vi "Get_user_id.vi"(8 "error in":errorcluster, 11 "Device In":T1) -> (0 "error out":errorcluster, 1 "id":string, 2 "Comm":T2, 3 "Device Out":T1)   [LabVIEW 2019]
uses:
  <userlib>/IoT Devices/_subVIs/HTTPComm.ctl
  <userlib>/Onshape/_SubVI/Cluster.ctl
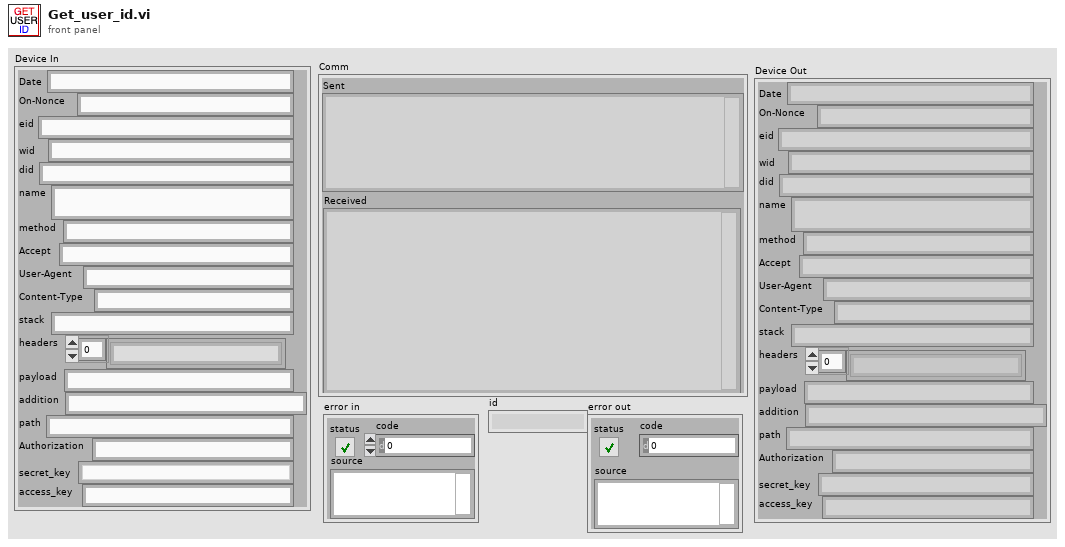
[diagram p1: front panel]
types:
  T1 = typedef "Cluster.ctl" = cluster{"Date":string, "On-Nonce":string, "eid":string, "wid":string, "did":string, "name":string, "method":string, "Accept":string, "User-Agent":string, "Content-Type":string, "stack":string, "headers":string[], "payload":string, "addition":string, "path":string, "Authorization":string, "secret_key":string, "access_key":string}
  T2 = typedef "HTTPComm.ctl" = cluster{"url":string, "sent headers":string, "sent body":string, "headers":string, "body":string, "Sent":string, "Received":string}
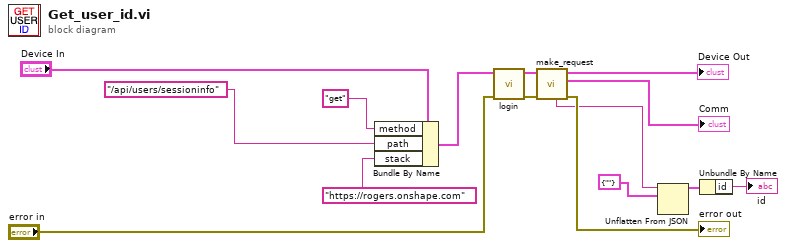
[diagram p0: block diagram]
diagram:
  n1 = Bundle By Name(cluster="Device In", "method"="get" ("Method"), "path"="/api/users/sessioninfo" ("payload"), "stack"="https://rogers.onshape.com" ("stacks")) -> (w6:T1)
  n2 = call <userlib>:"login.vi"("error in"="error in", "Device In"=w6) -> ("error out"=w10:errorcluster, "Device Out"=w13:T1)  [unwired: 8 in]
  n3 = call <userlib>:"make_request.vi"("Error in"=w10, "Device In"=w13) -> ("error out"=→"error out":errorcluster, "Comm"=→"Comm":T2, "Device Out"=→"Device Out":T1, "body"=w4:string)  [unwired: 5 in, 1 out]
  n4 = Unflatten From JSON(JSON string=w4, type and defaults=cluster{"id":string} {"id"=""}) -> (value=w2:cluster{"id":string})  [unwired: 5 in, 1 out]
  n5 = Unbundle By Name(w2) -> ("id"=→"id":string)
